vi "Dummy SubPanel.vi"(7 "Subpanel Event":refnum<user-event>) -> ()   [LabVIEW 2012, in "SubPanel.lvlib" / "SubPanel.lvclass"]
uses:
  SubPanel.lvclass
panel:
  in  "stop":bool
  in  "Transparency":dbl(slide) scale=0.0..80.0
  in  "Bkgd":u32(colorbox)=7171437
  out "Gauge":dbl(knob) scale=0.0..80.0
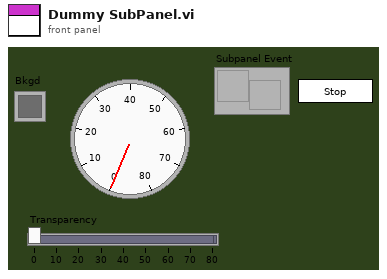
[diagram p1: front panel]
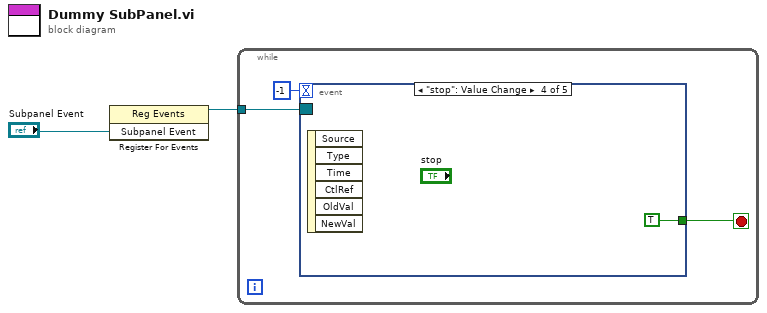
[diagram p0: block diagram]
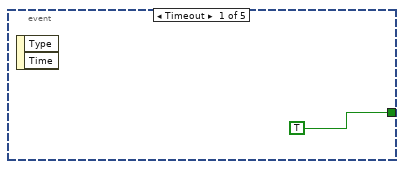
[diagram p2: hidden frame]
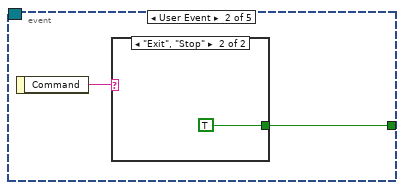
[diagram p3: hidden frame]
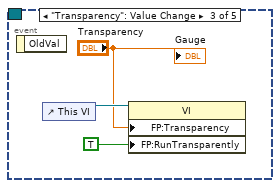
[diagram p5: hidden frame]
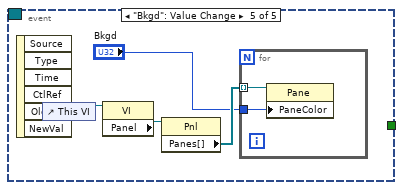
[diagram p6: hidden frame]
diagram:
  n1 = register-events("Subpanel Event") -> (reference out=w2:refnum<event-registration>)  [unwired: 2 in, 1 out]
  n2 = while {
    tunnel: w2 -> [w5]
    stop <- w3 stop-if-true
    n3 = event shown="[3] \"stop\": Value Change" {
      selector: w5 -> [_ _ _ _ _]
      dyn-events: _ -> [_ _ _ _ _]
      timeout: -1 -> [_ _ _ _ _]
      tunnel: [TRUE w7 _ TRUE _] -> w3
      event Timeout {
        n4 = event-data() -> ()  [unwired: 3 out]
      }
      event User Event {
        n5 = event-data() -> ("Command"=w8:string)  [unwired: 1 out]
        n6 = case shown="\"Exit\", \"Stop\"" w8 {
          tunnel: [_ TRUE] -> w7
          frame Default {
          }
          frame "Exit", "Stop" {
          }
        }
      }
      event "Transparency": Value Change {
        n7 = event-data() -> ()  [unwired: 2 out]
        n8 = control-ref of="This VI"() -> (w12:refnum<vi>)
        n9 = property class="VI"(reference=w12, "FP:Transparency"="Transparency", "FP:RunTransparently"=TRUE ("Front Panel Window:Run VI Transparently")) -> ()  [unwired: 1 in, 2 out]
        "Gauge" <- "Transparency"
      }
      event "stop": Value Change {
        n10 = event-data() -> ()  [unwired: 7 out]
      }
      event "Bkgd": Value Change {
        n11 = event-data() -> ()  [unwired: 7 out]
        n12 = control-ref of="This VI"() -> (w17:refnum<vi>)
        n13 = property class="VI"(reference=w17) -> ("Panel"=w16:refnum<vi>)  [unwired: 1 in, 2 out]
        n14 = property class="Pnl"(reference=w16) -> ("Panes[]"=w15:refnum<vi>[])  [unwired: 1 in, 2 out]
        n15 = for {
          tunnel: w15 -> [w19] mode=indexing
          tunnel: "Bkgd" -> [w18]
          n16 = property class="Pane"(reference=w19, "PaneColor"=w18) -> ()  [unwired: 1 in, 2 out]
        }
      }
    }
  }
